vi "DEM2.vi"(8 "error in (no error)":errorcluster, 10 "input":cdb[](array[numeric]), 11 "Frame Instruction 3":T1={"Code Rates"=4.0, "Length"=12.0, "Destination address"=8.0, "User"=2.0, "Source address "=12.0, " Frame number"=8.0, "Check Sum"=16.0}) -> (0 "error out":errorcluster, 2 "output bit stream":i8[](array[numeric]), 3 "Frame":i32)   [LabVIEW 2014]
uses:
  <vilib>/addons/Modulation/Digital/General/MT Map PSK Symbols to Bits.vi
  <vilib>/addons/Modulation/Digital/General/MT Map QAM Symbols to Bits.vi
  <vilib>/addons/Modulation/Digital/General/MT Generate QAM System Parameters(M).vi
  <vilib>/addons/Modulation/niDMT.lvlib
panel:
  out "Array 5":u32[](array[numeric])
  out "Array 4":i8[][](array[numeric])
  out "size(s)":i32
  out "Array":bool[](array[boolean])
  out "16QAM":cdb[](graph)
  out "4QAM":cdb[](graph)
  out "BSPK Data":cdb[](graph)
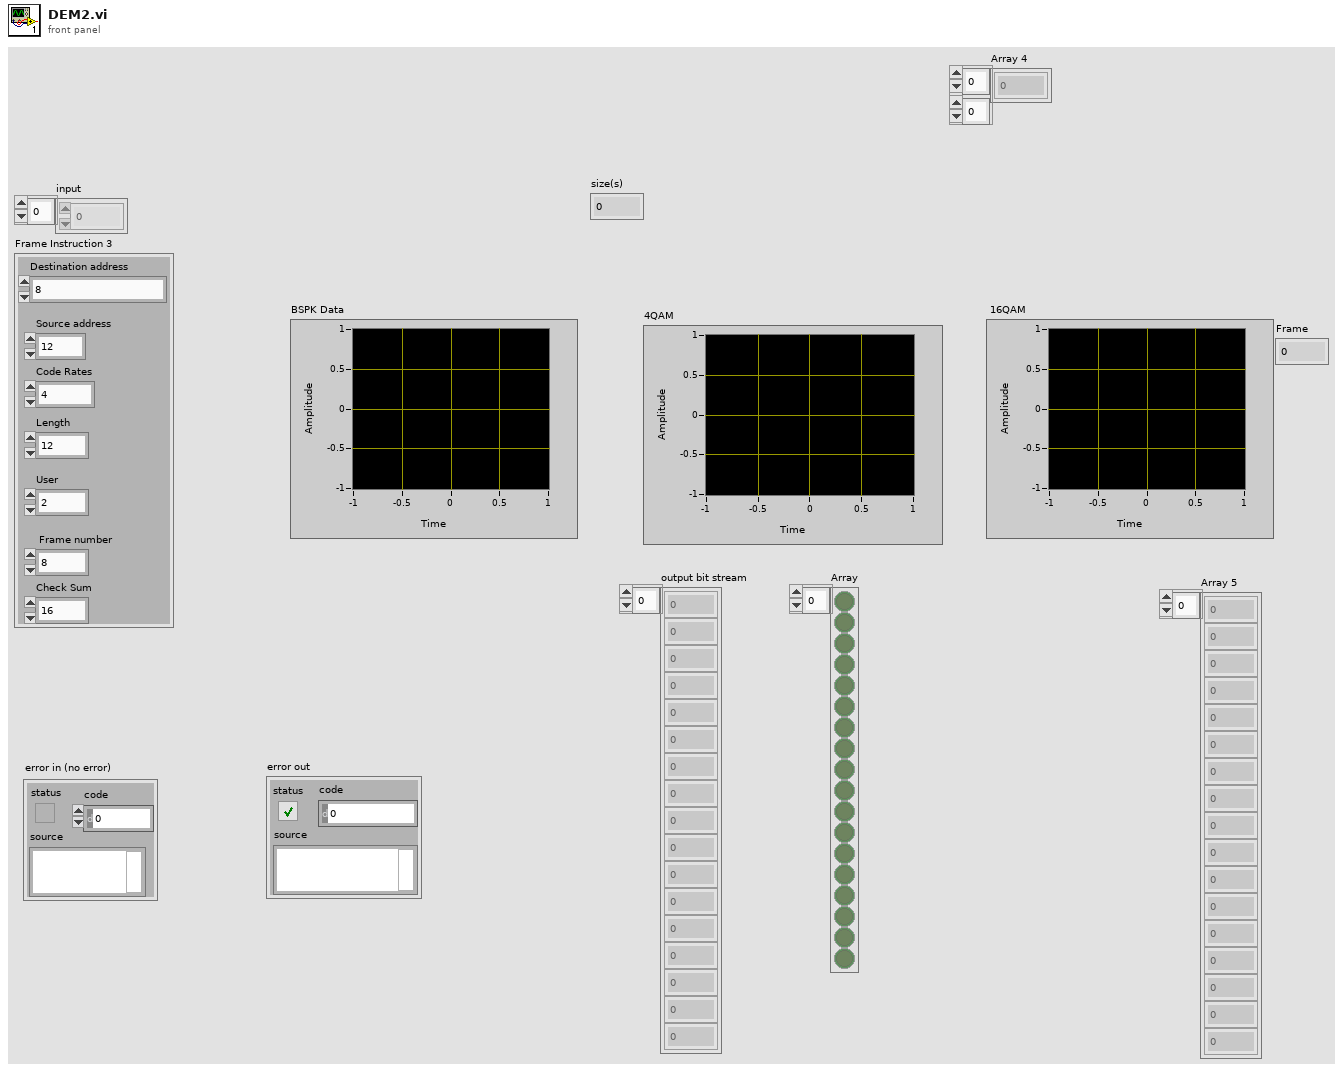
[diagram p1: front panel]
types:
  T1 = cluster{"Code Rates":dbl, "Length":dbl, "Destination address":dbl, "User":dbl, "Source address ":dbl, " Frame number":dbl, "Check Sum":dbl}
  T2 = cluster{"samples per symbol (16)":i32, "symbol map":cdb[]}
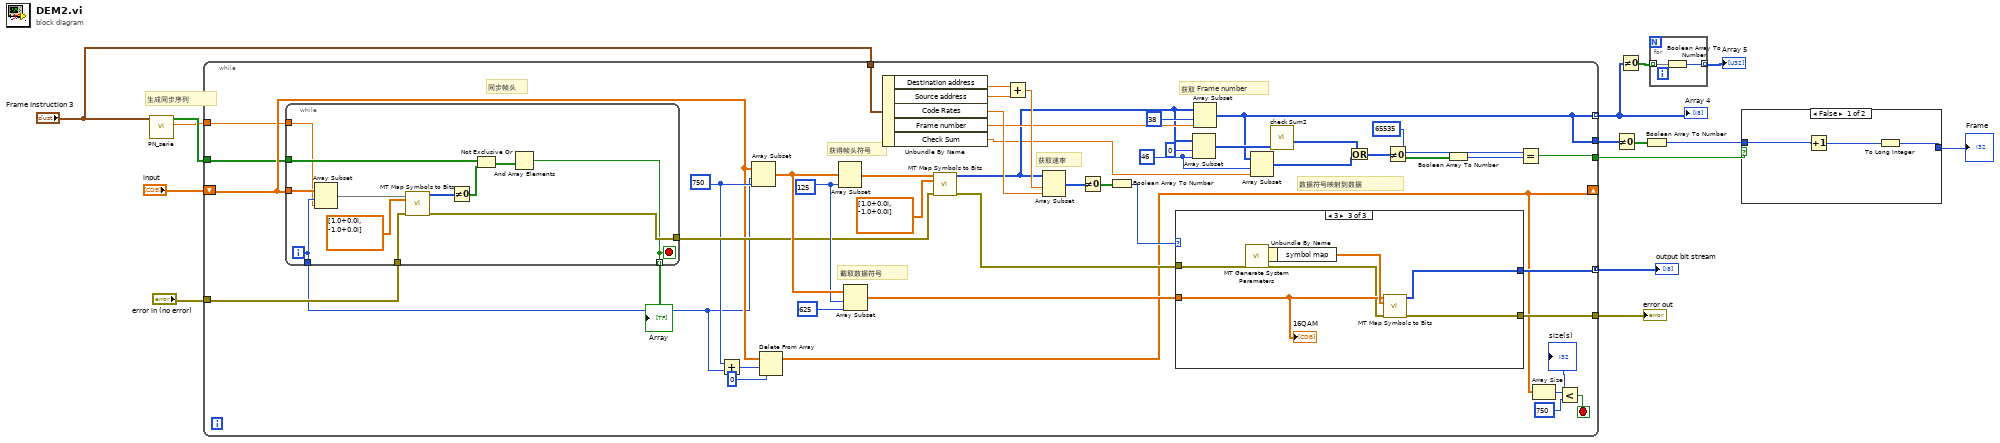
[diagram p0: block diagram]
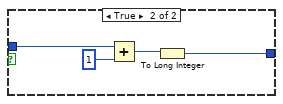
[diagram p2: hidden frame]
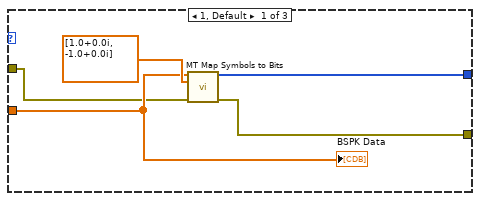
[diagram p3: hidden frame]
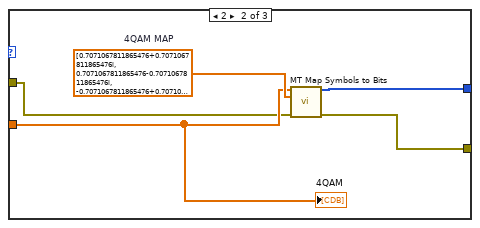
[diagram p4: hidden frame]
diagram:
  # "生成同步序列"
  n1 = call "PN_serie.vi"("Frame Instruction 3"="Frame Instruction 3") -> ("同步大小"=w6:dbl, "同步序列"=w7:bool[])  [unwired: 9 in]
  n2 = while {
    tunnel: "error in (no error)" -> [w61]
    tunnel: "Frame Instruction 3" -> [w60]
    tunnel: [w46] -> w12 mode=concatenating
    tunnel: [w43] -> w13
    shift-right: [w32] -> _
    shift-left: "input" -> [w34]
    tunnel: [w25] -> w11 mode=indexing
    tunnel: [w25] -> w4
    tunnel: w7 -> [w30]
    tunnel: w6 -> [w29]
    tunnel: [w18] -> w5
    stop <- w38 stop-if-true
    w24 = 46
    w58 = 125
    w41 = 750
    # "获取 Frame number"
    # "获取速率"
    # "数据符号映射到数据"
    # "截取数据符号"
    # "获得帧头符号"
    # "同步帧头"
    n3 = while {
      tunnel: w34 -> [w90]
      tunnel: w61 -> [w87]
      tunnel: [w83] -> w33
      tunnel: [w82] -> w45
      tunnel: [w81] -> w35 mode=indexing
      tunnel: w30 -> [w80]
      tunnel: w29 -> [w79]
      i -> [w83]
      stop <- w81 stop-if-true
      n4 = Array Subset(array=w90, index=w83, length=w79) -> (w89:cdb[])
      n5 = call-poly <vilib>:"MT Map Symbols to Bits.vi"("symbols"=w89, "symbol map"=cdb[] [1.0+0.0i, -1.0+0.0i], "error in (no error)"=w87) -> ("output bit stream"=w86:i8[], "error out"=w82:errorcluster)  [unwired: 11 in]
      n6 = Not Equal To 0?(x=w86) -> (x != 0?=w85:bool[])
      n7 = Not Exclusive Or(1:w85, 2:w80) -> (0:w84:bool[])
      n8 = And Array Elements(Boolean array=w84) -> (logical AND=w81:bool)
    }
    "Array" <- w35
    n9 = Add(x=w41, y=w33) -> (x+y=w42:i32)
    n10 = Array Subset(array=w34, index=w33, length=w41) -> (w59:cdb[])
    n11 = Delete From Array(array=w34, length=w42, index=0) -> (array with subset deleted=w32:cdb[])  [unwired: 1 out]
    n12 = Array Subset(array=w59, length=w58) -> (w55:cdb[])  [unwired: 1 in]
    n13 = Array Subset(array=w59, index=w58, length=625) -> (w56:cdb[])
    n14 = Unbundle By Name(w60) -> ("Destination address"=w53:dbl, "Source address"=w52:dbl, "Code Rates"=w50:dbl, "Frame number"=w37:dbl, "Check Sum"=w23:dbl)
    n15 = call-poly <vilib>:"MT Map Symbols to Bits.vi"("symbols"=w55, "symbol map"=cdb[] [1.0+0.0i, -1.0+0.0i], "error in (no error)"=w45) -> ("output bit stream"=w28:i8[], "error out"=w44:errorcluster)  [unwired: 11 in]
    n16 = Add(x=w53, y=w52) -> (x+y=w51:dbl)
    n17 = Array Subset(array=w28, index=w51, length=w50) -> (w49:i8[])
    n18 = Not Equal To 0?(x=w49) -> (x != 0?=w48:bool[])
    n19 = Boolean Array To Number(Boolean array=w48) -> (number=w47:u32)
    n20 = case shown="3" w47 {
      tunnel: w56 -> [w64 w70 w75]
      tunnel: [w65 w69 w76] -> w46
      tunnel: w44 -> [w63 w68 w74]
      tunnel: [w62 w67 w72] -> w43
      frame 1, Default {
        n21 = call-poly <vilib>:"MT Map Symbols to Bits.vi"("symbols"=w64, "symbol map"=cdb[] [1.0+0.0i, -1.0+0.0i], "error in (no error)"=w63) -> ("output bit stream"=w65:i8[], "error out"=w62:errorcluster)  [unwired: 11 in]
        "BSPK Data" <- w64
      }
      frame 2 {
        w71 = cdb[] [0.7071067811865476+0.7071067811865476i, 0.7071067811865476-0.7071067811865476i, -0.7071067811865476+0.7071067811865476i, -0.7071067811865476-0.7071067811865476i]  # 4QAM MAP
        n22 = call-poly <vilib>:"MT Map Symbols to Bits.vi"("symbols"=w70, "symbol map"=w71, "error in (no error)"=w68) -> ("output bit stream"=w69:i8[], "error out"=w67:errorcluster)  [unwired: 11 in]
        "4QAM" <- w70
      }
      frame 3 {
        n23 = call-poly <vilib>:"MT Generate System Parameters.vi"("error in (no error)"=w74) -> ("QAM system parameters"=w78:T2, "error out"=w73:errorcluster)  [unwired: 12 in, 1 out]
        n24 = Unbundle By Name(w78) -> ("symbol map"=w77:cdb[])
        n25 = call-poly <vilib>:"MT Map Symbols to Bits.vi"("symbols"=w75, "symbol map"=w77, "error in (no error)"=w73) -> ("output bit stream"=w76:i8[], "error out"=w72:errorcluster)  [unwired: 11 in]
        "16QAM" <- w75
      }
    }
    n26 = Array Subset(array=w28, index=0, length=w24) -> (w26:i8[])
    n27 = Array Subset(array=w28, index=38, length=w37) -> (w25:i8[])
    n28 = Array Subset(array=w25, index=w24, length=w23) -> (w21:i8[])
    n29 = call "check Sum2.vi"("Array"=w26) -> ("subarray"=w22:i16[])  [unwired: 10 in]
    n30 = Or(x=w22, y=w21) -> (x .or. y?=w20:i16[])
    n31 = Not Equal To 0?(x=w20) -> (x != 0?=w17:bool[])
    n32 = Boolean Array To Number(Boolean array=w17) -> (number=w16:u32)
    n33 = Equal?(x=65535, y=w16) -> (x = y?=w18:bool)
    n34 = Array Size(array=w32) -> (size(s)=w40:i32)
    "size(s)" <- w40
    n35 = Less?(x=w40, y=750) -> (x < y?=w38:bool)
  }
  "output bit stream" <- w12
  "error out" <- w13
  "Array 4" <- w11
  n36 = Not Equal To 0?(x=w4) -> (x != 0?=w3:bool[])
  n37 = Not Equal To 0?(x=w11) -> (x != 0?=w10:bool[][])
  n38 = Boolean Array To Number(Boolean array=w3) -> (number=w2:u32)
  n39 = for {
    tunnel: w10 -> [w92] mode=indexing
    tunnel: [w91] -> w9 mode=indexing
    n40 = Boolean Array To Number(Boolean array=w92) -> (number=w91:u32)
  }
  "Array 5" <- w9
  n41 = case shown="False" w5 {
    tunnel: w2 -> [w94 w99]
    tunnel: [w95 w96] -> w1
    frame False {
      n42 = Increment(x=w94) -> (x+1=w93:u32)
      n43 = To Long Integer(number=w93) -> (32bit integer=w95:i32)
    }
    frame True {
      n44 = Add(x=w99, y=1) -> (x+y=w97:u32)
      n45 = To Long Integer(number=w97) -> (32bit integer=w96:i32)
    }
  }
  "Frame" <- w1
